vi "Update Details.vi"(8 "error in (no error)":errorcluster, 10 "event data":refnum<class "Generic Item.lvclass">, 11 "Instrument In":refnum<class "Instrument.lvclass">) -> (0 "error out":errorcluster, 3 "Instrument Out":refnum<class "Instrument.lvclass">)   [LabVIEW 2015, in "Item Actor.lvlib" / "Instrument.lvclass"]
uses:
  Instrument.lvclass
  Generic Item/Generic Item.lvclass
  Instrument.lvclass/Instrument.ctl
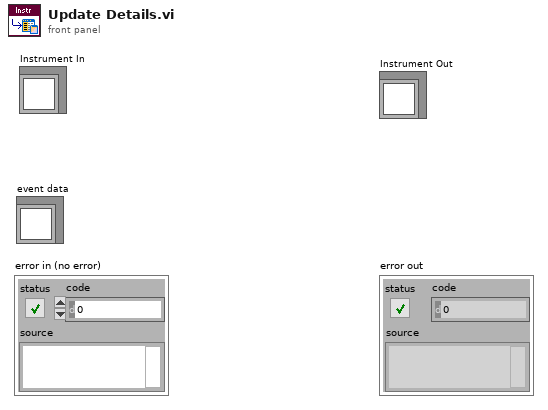
[diagram p1: front panel]
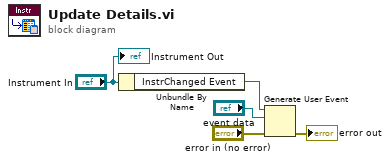
[diagram p0: block diagram]
diagram:
  n1 = Unbundle By Name("Instrument In") -> ("InstrChanged Event"=w2:refnum<user-event>)
  n2 = Generate User Event(user event=w2, event data cluster="event data", error in="error in (no error)") -> (error out=→"error out":errorcluster)  [unwired: 1 in, 1 out]
  "Instrument Out" <- "Instrument In"
